vi "temperture.vi"() -> ()   [LabVIEW 2010]
panel:
  in  "Temperature In":dbl format="%.2f"
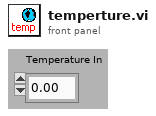
[diagram p1: front panel]
diagram:
